vi "MES_Get Parameters.vi"(0 "Name":string, 1 "Order By":T1, 5 "Main":string, 9 "VariableName":string, 11 "error in (no error)":errorcluster, 12 "Alarm":bool=TRUE) -> (2 "FirstRow":string[](array[string]), 3 "Value1 List":string[](array[string]), 4 "Value 1":T2, 6 "Value  2":T2, 8 "Value  3":T2, 10 "Unit":string, 13 "First row value list":string[](array[string]), 14 "Table Control 2":string[][](table), 15 "error out":errorcluster)   [LabVIEW 2021, in "SQLite.lvclass"]
doc: "读取MES与PLC通讯的IP地址，DB块，DBB地址，format\n# 2020-5-13 13:25:16\n# daikinyi\n蒋松\njiangsong@outlook.com"
uses:
  SQLite.lvclass
  Control/value Type.ctl
  Order By.ctl
  TabelFullName.ctl
  SQLiteFileName.ctl
  <userlib>/LabSQL/LabSQL.lvlib
  <userlib>/sushu/sushu.lvlib
panel:
  out "formatList":string[](array[string])
  out "PLC DB DBBList":string[](array[string])
  out "number (0 to 1)":dbl
  out "Select SQL CMD":string
  # "组装线体的编号"
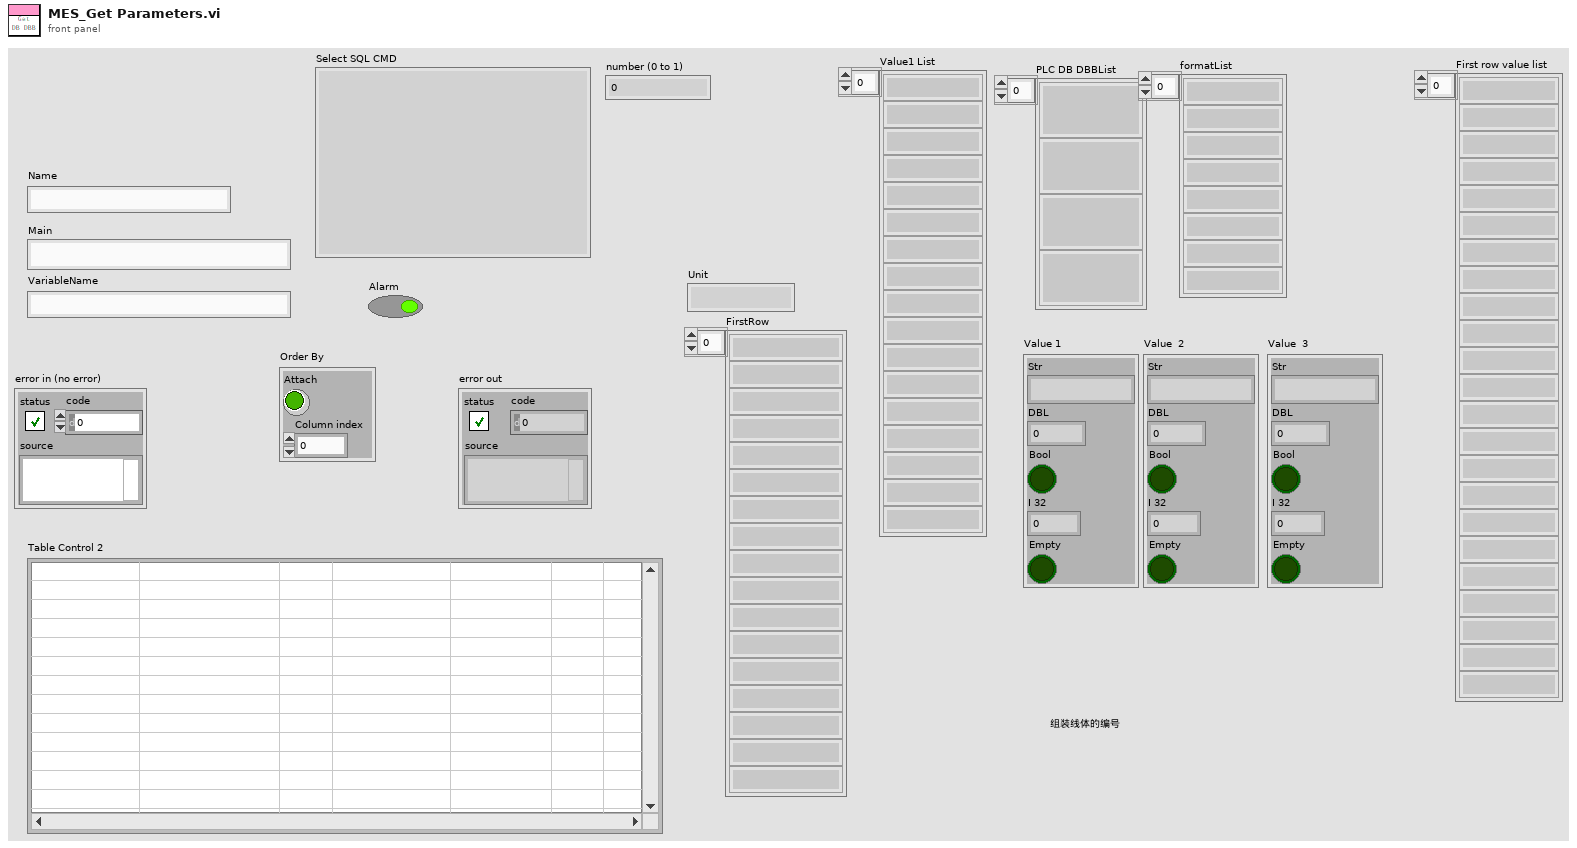
[diagram p1: front panel]
types:
  T1 = typedef "SQLite.lvclass/Order By.ctl" = cluster{"Attach":bool, "Column index":i32}
  T2 = typedef "SQLite.lvclass/value Type.ctl" = cluster{"Str":string, "DBL":dbl, "Bool":bool, "I 32":i32, "Empty":bool}
  T3 = enum16{"Initialize", "Read", "Write", "UnInitialize"}
  T4 = typedef "SQLite.lvclass/TabelFullName.ctl" = string
  T5 = cluster{"Current VI Reference":refnum<vi>, "Close Panel on Exit?":bool}
  T6 = cluster{"Core":cluster{"Current VI Reference":refnum<vi>, "Close Panel on Exit?":bool}, "VI Name":string}
  T7 = typedef "SQLite.lvclass/SQLiteFileName.ctl" = string
  T8 = enum16{"Other", "SQL2008", "SQLite", "Access", "MySQL"}
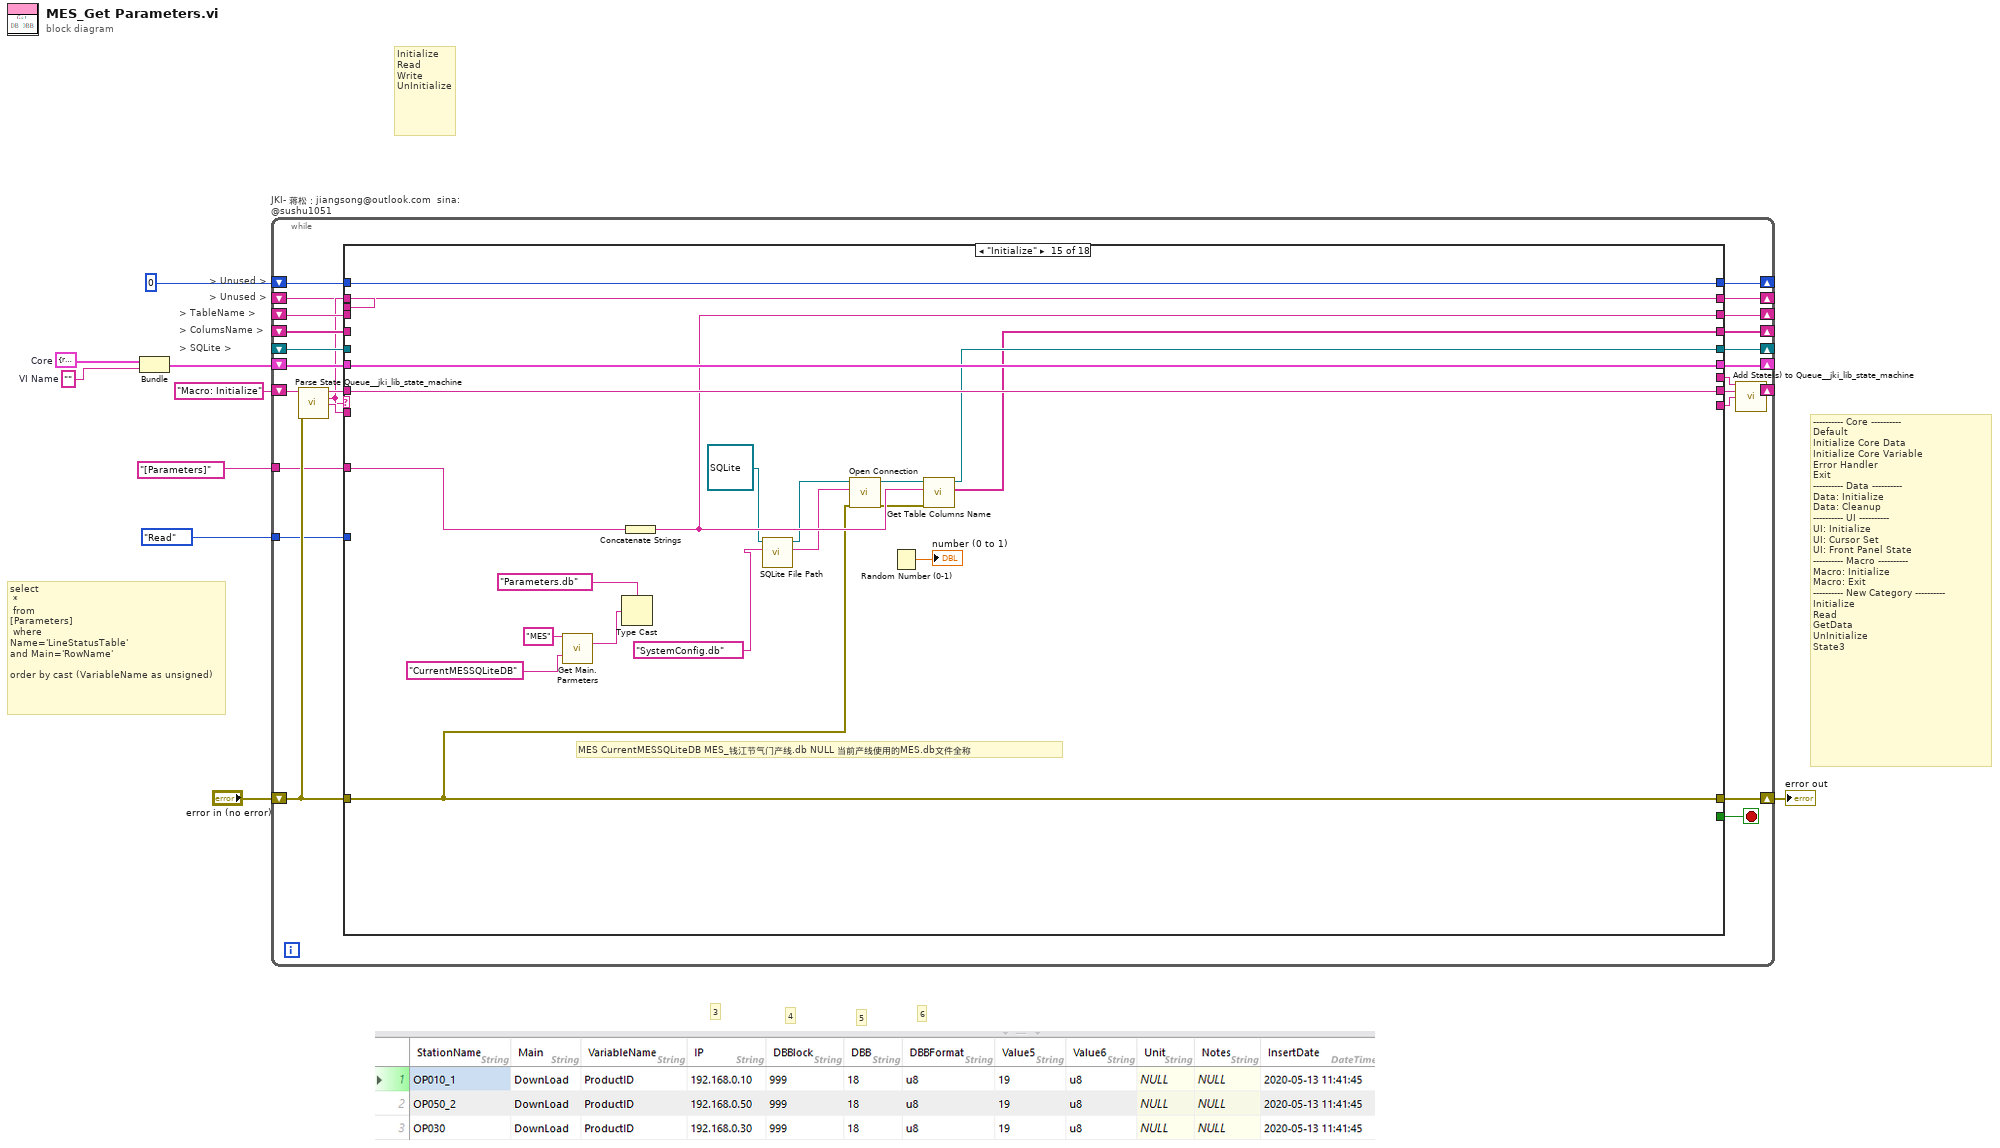
[diagram p0: block diagram]
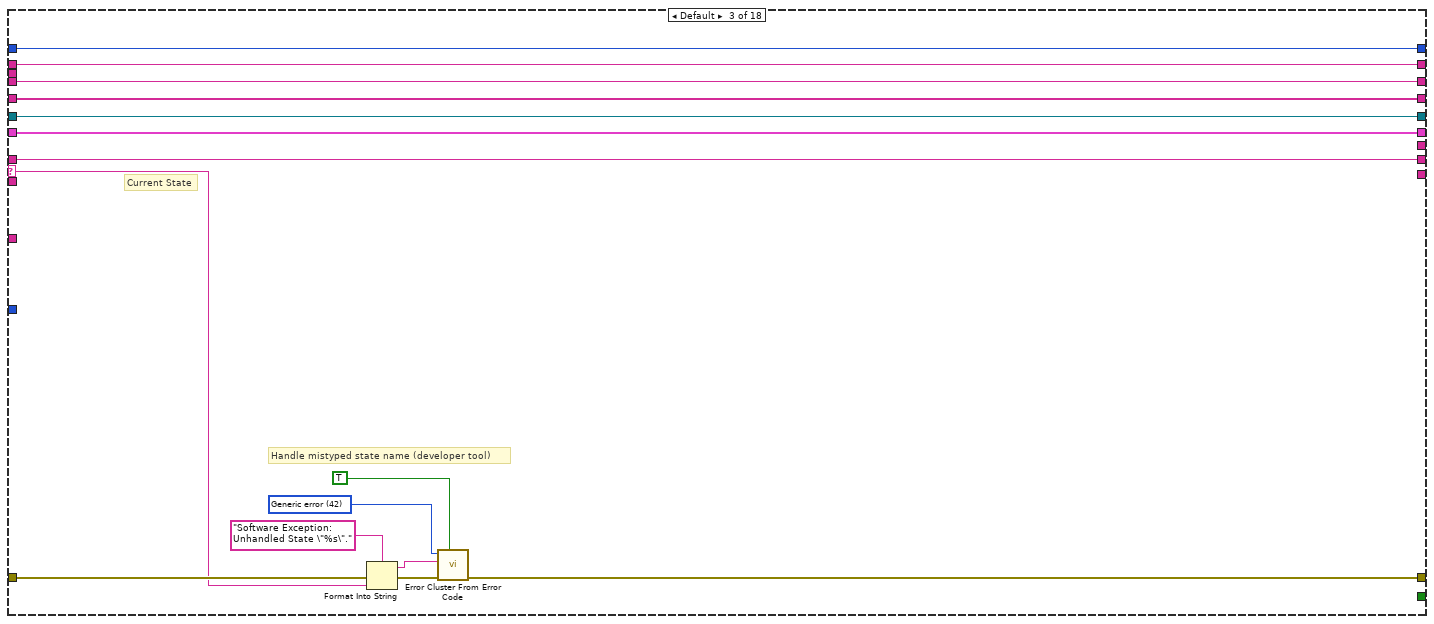
[diagram p4: hidden frame]
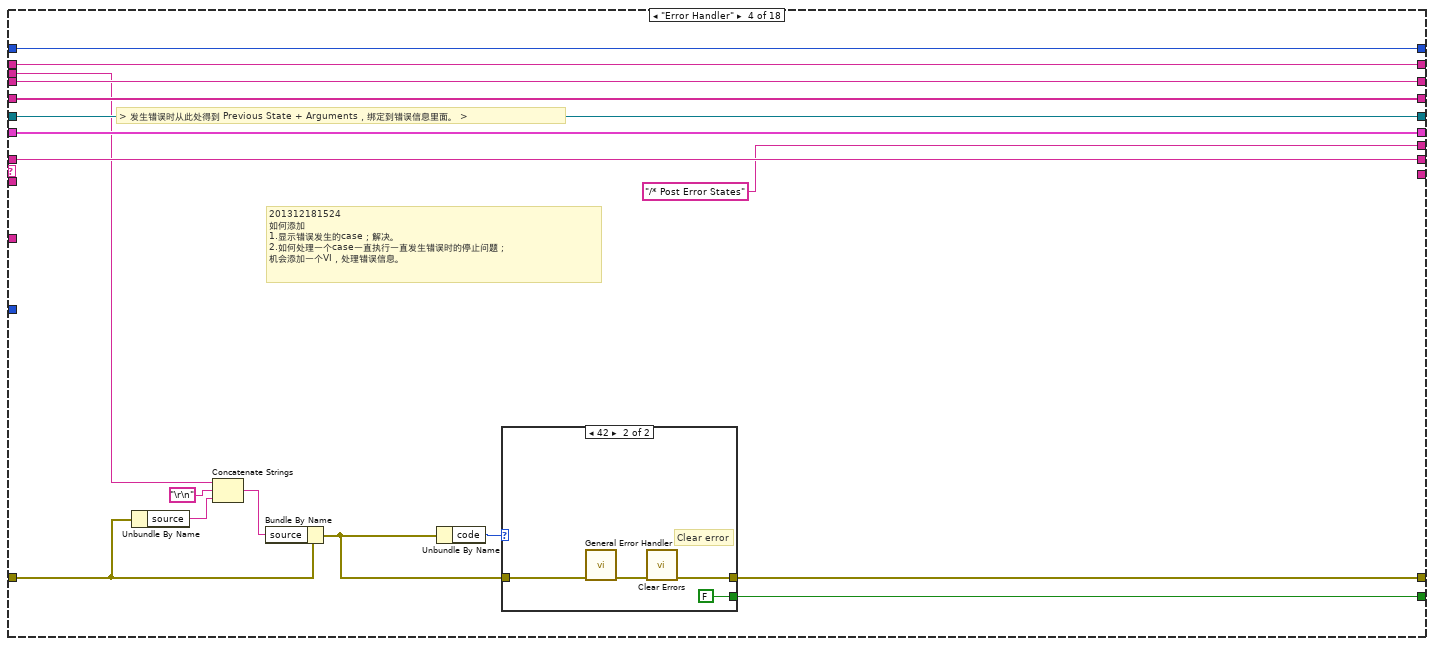
[diagram p5: hidden frame]
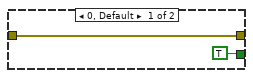
[diagram p6: hidden frame]
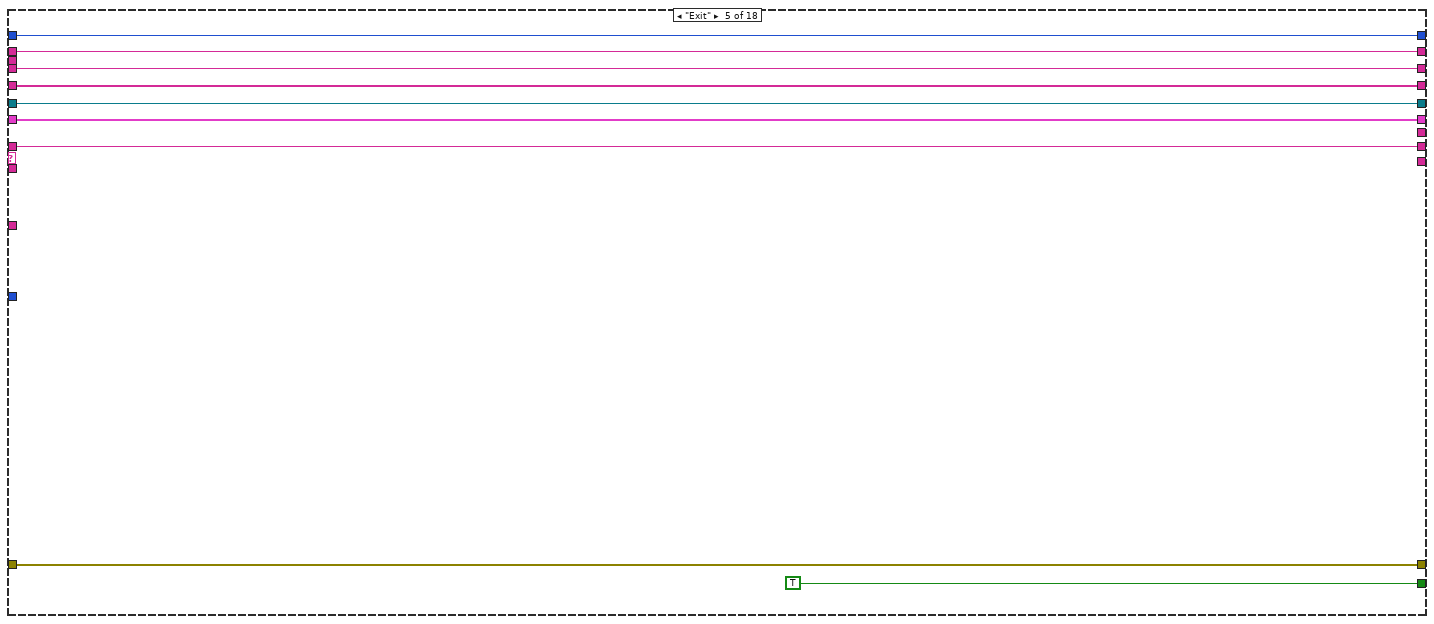
[diagram p7: hidden frame]
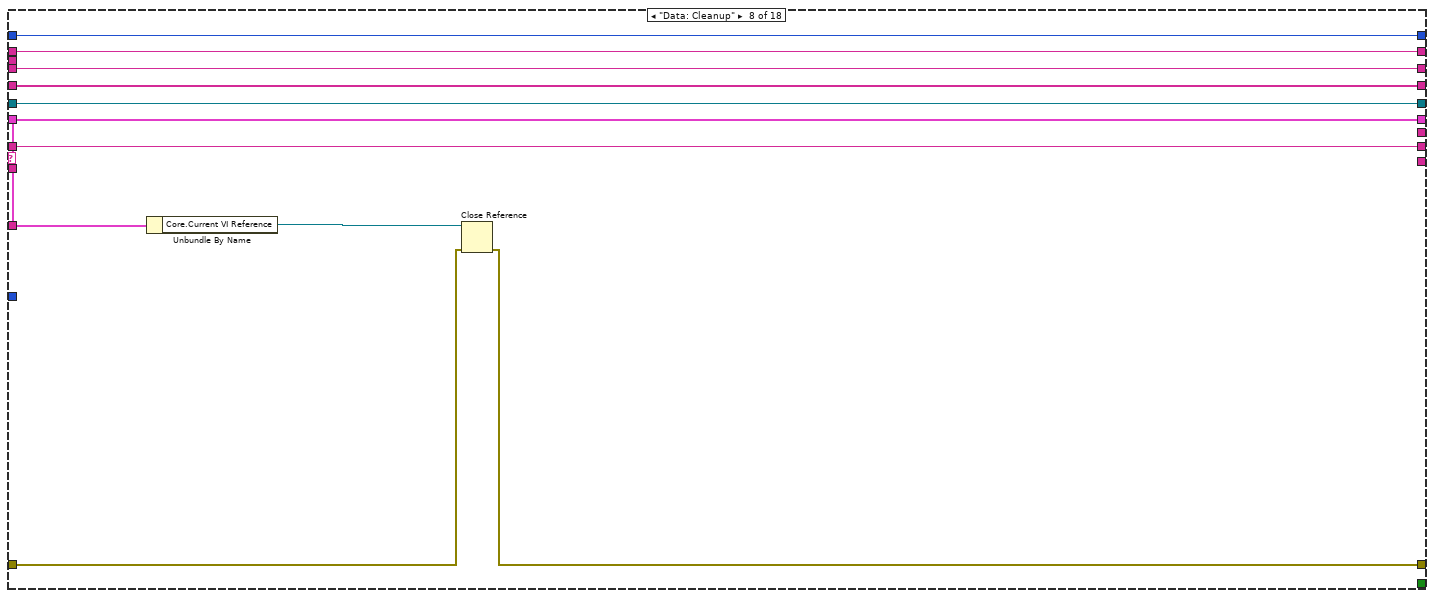
[diagram p10: hidden frame]
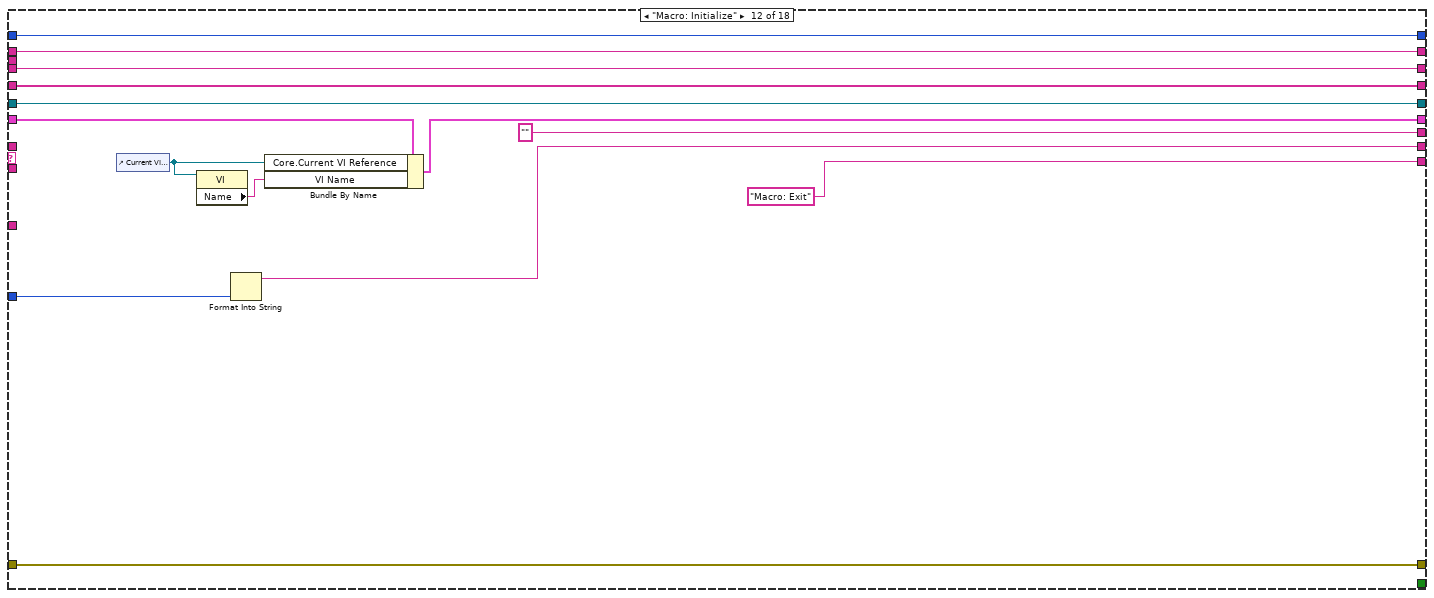
[diagram p14: hidden frame]
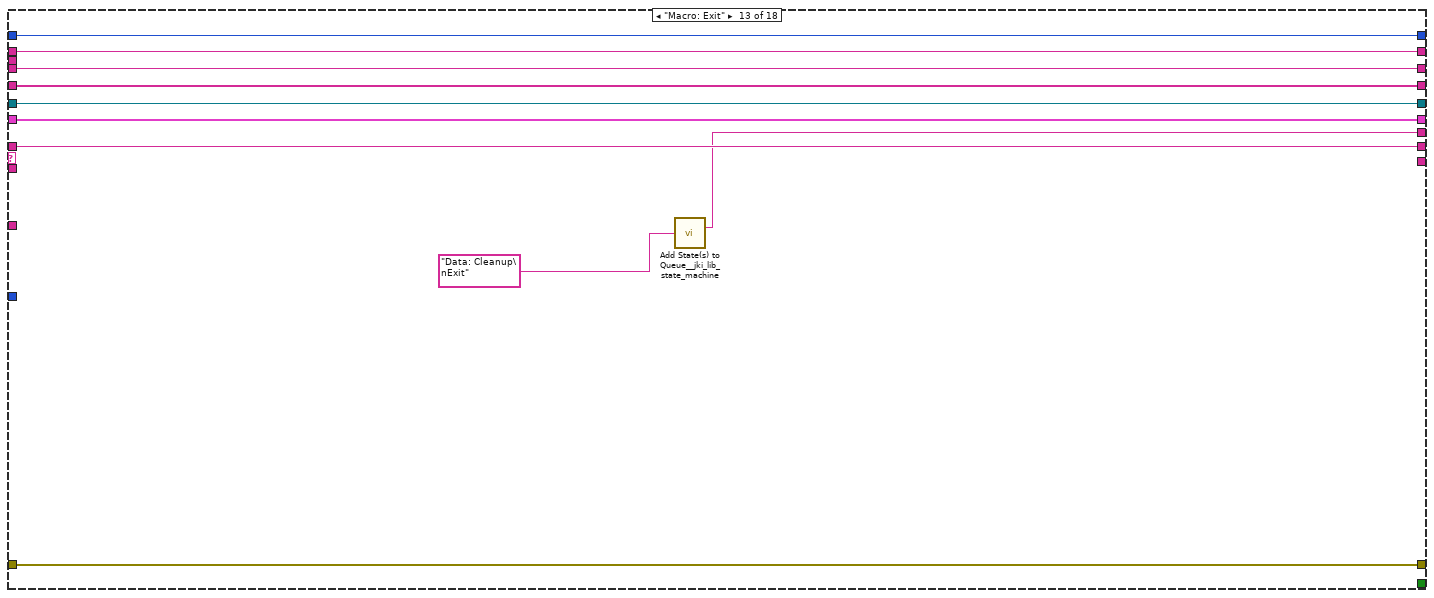
[diagram p15: hidden frame]
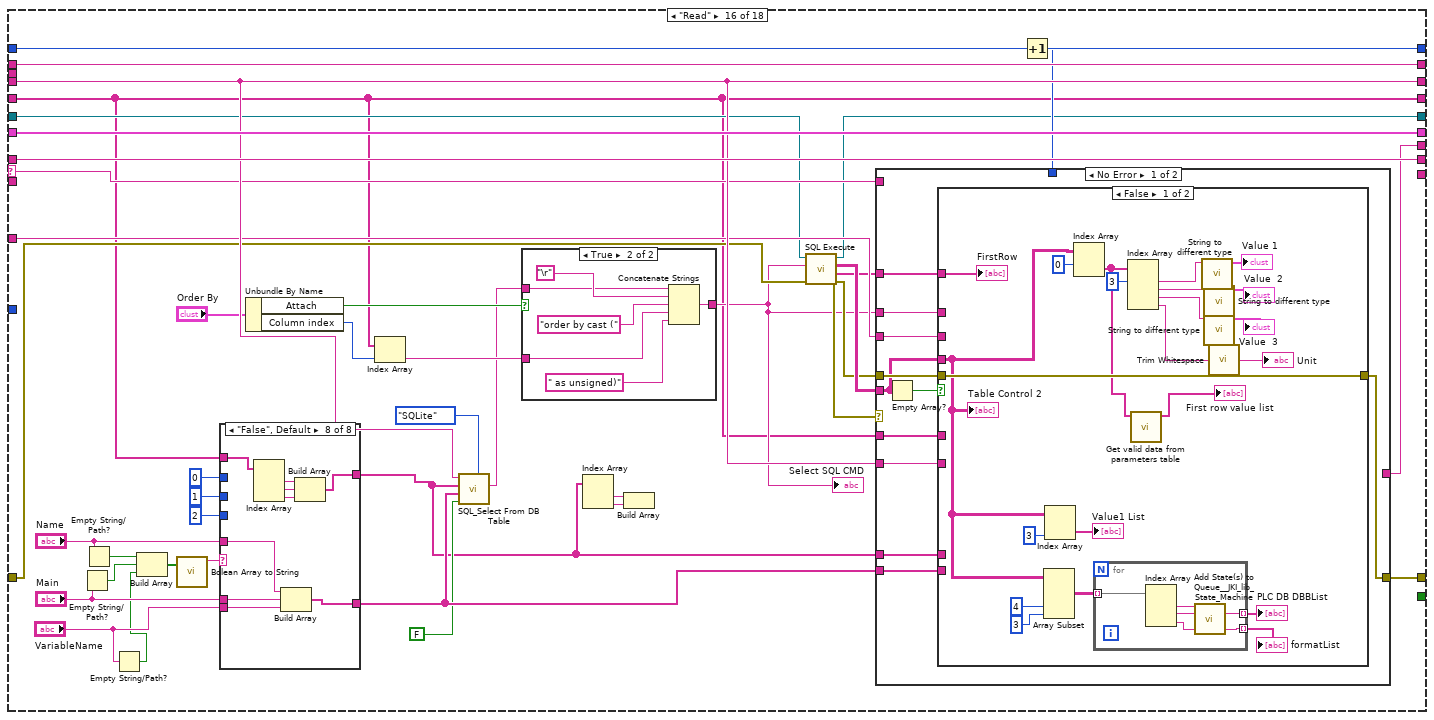
[diagram p17: hidden frame]
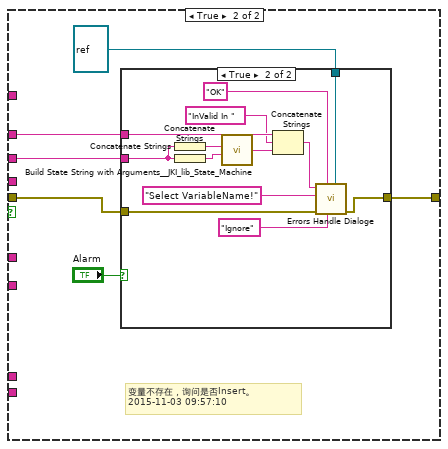
[diagram p19: hidden frame]
diagram:
  w9 = ""  # VI Name
  w8 = T5 {"Current VI Reference"=refnum, "Close Panel on Exit?"=FALSE}  # Core
  # "select \n * \n from \n[Parameters]\n where \nName='LineStatusTable'\nand Main='RowName'\n\norder by cast (VariableName as unsigned)"
  # "6"
  # "5"
  # "4"
  # "3"
  # "Initialize\nRead\nWrite\nUnInitialize"
  # "> Unused >"
  # "> SQLite >"
  # "> ColumsName >"
  # "> TableName >"
  # "> Unused >"
  # "---------- Core ----------\nDefault\nInitialize Core Data\nInitialize Core Variable\nError Handler\nExit\n---------- Data ----------\nData: Initialize\nData: Cleanup\n---------- UI ----------\nUI: Initialize\nUI: Cursor Set\nUI: Front Panel State\n---------- Macro ----------\nMacro: Initialize\nMacro: Exit\n---------- New Category ----------\nInitialize\nRead\nGetData\nUnInitialize\nState3"
  n1 = Bundle("Core"=w8, "VI Name"=w9) -> (w7:T6)  [unwired: 1 in]
  n2 = while "JKI- 蒋松：jiangsong@outlook.com  sina: @sushu1051" {
    shift-right: [w32] -> w2
    shift-left: "error in (no error)" -> [w30]
    shift-right: [w20] -> _
    shift-left: "Macro: Initialize" -> [w21]
    shift-right: [w27] -> _
    shift-left: _ -> [w29]
    shift-right: [w28] -> _
    shift-left: _ -> [w10]
    shift-right: [w22] -> _
    shift-left: w7 -> [w25]
    shift-right: [w23] -> _
    shift-left: _ -> [w16]
    shift-right: [w24] -> _
    shift-left: _ -> [w26]
    shift-right: [w15] -> _
    shift-left: 0 -> [w14]
    tunnel: T3."Read" ("CMD") -> [w13]
    tunnel: T4 "[Parameters]" ("TabelFullName") -> [w12]
    stop <- w31 stop-if-true
    n3 = call <vilib>:"Parse State Queue__jki_lib_state_machine.vi"("State Queue"=w21, "Error In (no error)"=w30) -> ("Remaining States"=w34:string, "Current State"=w11:string, "Arguments"=w33:string)  [unwired: 10 in, 1 out]
    n4 = case shown="\"Initialize\"" w11 {
      selector: w11 -> [_ _ w53 _ _ _ _ _ _ _ _ _ _ _ _ w230 _ _]
      tunnel: w34 -> [w42 w44 w52 w74 w90 w99 w108 w115 w125 w133 w141 _ w164 w173 w199 w239 w386 w396]
      tunnel: w33 -> [_ _ _ _ _ _ _ _ _ _ _ _ _ _ _ _ _ _]
      tunnel: [w41 w50 w54 w68 w92 w101 w110 w117 w127 w135 w143 w158 w168 w176 w189 w231 w379 w387] -> w32
      tunnel: w30 -> [w41 w50 w55 w78 w92 w101 w110 w118 w127 w135 w143 w158 w168 w176 w189 w224 w379 w388]
      tunnel: [w42 w44 w52 w74 w90 w99 w108 w115 w125 w133 w141 w149 w164 w173 w199 w239 w386 w396] -> w19
      tunnel: [_ _ _ w67 TRUE _ _ _ _ _ _ _ _ _ _ _ _ _] -> w31
      tunnel: w11 -> [w40 w49 w65 w82 w97 w105 w113 w123 w131 w139 w147 w161 w171 w179 w198 w232 w380 w395]
      tunnel: w29 -> [w39 w48 w64 w81 w96 w104 w112 w122 w130 w138 w146 w160 w170 w178 _ w234 w385 w394]
      tunnel: [w40 w49 w65 w82 w97 w105 w113 w123 w131 w139 w147 w161 w171 w179 w198 w232 w380 w395] -> w28
      tunnel: [w39 w48 w64 w81 w96 w104 w112 w122 w130 w138 w146 w160 w170 w178 w191 w234 w385 w394] -> w27
      tunnel: w26 -> [w38 w47 w63 w80 w95 w103 w111 w121 w129 w137 w145 w159 w169 w177 _ w206 w384 w393]
      tunnel: w16 -> [w36 w45 w62 w72 w91 w100 w109 w116 w126 w134 w142 w157 w165 w174 _ w227 w383 w390]
      tunnel: w25 -> [w37 w46 w61 w79 w94 w102 w106 w119 w128 w136 w144 w151 w166 w175 w197 w238 w382 w392]
      tunnel: [w38 w47 w63 w80 w95 w103 w111 w121 w129 w137 w145 w159 w169 w177 w192 w206 w384 w393] -> w24
      tunnel: [w36 w45 w62 w72 w91 w100 w109 w116 w126 w134 w142 w157 w165 w174 w193 w225 w383 w389] -> w23
      tunnel: [w37 w46 w61 w79 w94 w102 w106 w119 w128 w136 w144 w150 w166 w175 w197 w238 w382 w392] -> w22
      tunnel: [_ _ _ "/* Post Error States" _ _ _ _ _ _ _ "" w163 _ _ w229 _ _] -> w18
      tunnel: [_ _ _ _ _ _ _ _ _ _ _ "Macro: Exit" _ _ _ _ _ _] -> w17
      tunnel: w14 -> [w35 w43 w51 w71 w89 w98 w107 w114 w124 w132 w140 w156 w162 w172 w196 w228 w381 w391]
      tunnel: [w35 w43 w51 w71 w89 w98 w107 w114 w124 w132 w140 w156 w162 w172 w196 w237 w381 w391] -> w15
      tunnel: w13 -> [_ _ _ _ _ _ _ _ _ _ _ w148 _ _ _ _ _ _]
      tunnel: w12 -> [_ _ _ _ _ _ _ _ _ _ _ _ _ _ w194 w233 _ _]
      tunnel: w10 -> [_ _ _ w66 _ _ _ _ _ _ _ _ _ _ _ _ _ _]
      frame "Idle" {
      }
      frame "---------- Core ----------" {
      }
      frame Default {
        w57 = 42 items=["No error", "Argument error", "Memory is full", "Out of zone", "End of file", "File already open", "Generic file I/O error", "File not found", "File permission error", "Disk is full", "Duplicate path", "Too many files open", "System feature not enabled", "Resource file not found", "Cannot add resource", "Resource not found", "Image not found", "Image memory error", "Pen does not exist", "Config type invalid", "Config token not found", "Config parse error", "Config memory error", "Bad external code format", "Bad external code offset", "External code not present", "Null window", "Destroy window error", "Null menu", "Print aborted", "Bad print record", "Print driver error", "Windows error during printing", "Memory error during printing", "Print dialog error", "Generic print error", "Invalid device refnum", "Device not found", "Device parameter error", "Device unit error", "Cannot open device", "Device call aborted", "Generic error", "Cancelled by user", "Object ID too low", "Object ID too high", "Object not in heap", "Unknown heap", "Unknown object (invalid DefProc)", "Unknown object (DefProc not in table)", "Message out of range", "Invalid (null) method", "Unknown message", "Manager call not supported", "Bad address", "Network operation in progress", "Network operation timed out", "Connection is busy", "Network attribute not supported", "Network error", "Address in use", "System out of memory", "Connection aborted", "Connection refused", "Not connected", "Already connected", "Connection closed", "Initialization error (interapplication manager)", "Bad occurrence", "Wait on unbound occurrence handler", "Occurrence queue overflow", "Datalog type conflict", "Unused", "Unrecognized type (interapplication manager)", "Memory corrupt", "Failed to make temporary DLL", "Old CIN version", "Drag socket not found", "Failed to load drop-object", "Failed to register OLE object", "Failed to release OLE object", "Format specifier type mismatch", "Unknown format specifier", "Too few format specifiers", "Too many format specifiers", "Scan failed", "Newer CIN version", "Error converting to variant", "Runtime menu error", "Password tampered", "Variant attribute not found", "Incompatible variant data type", "Event data is not available", "Event Store is not present", "Occurrence is not found", "Event Queue is not created", "Event info is not available", "Refnum passed is NULL", "Error retrieving Class GUID", "Error retrieving CoClass GUID", "Error retrieving TypeLib GUID.", "Bad built application magic bytes.", "Specific driver is different from the specific driver associated with the Logical Name.", "There is no session opened to the class driver.", "Max Error", "MAX - Error with config objects", "MAX - Error loading configuration", "MAX - Group not supported"]
        # "Current State"
        # "Handle mistyped state name (developer tool)"
        n5 = Format Into String(format string="Software Exception: Unhandled State \"%s\"." ("message"), error in=w55, w53) -> (resulting string=w58:string, error out=w59:errorcluster)  [unwired: 1 in]
        n6 = call <vilib>:"Error Cluster From Error Code.vi"("show call chain? (False)"=TRUE, "error in (no error)"=w59, "error message (\"\")"=w58, "error code (0)"=w57) -> ("error out"=w54:errorcluster)  [unwired: 5 in]
      }
      frame "Error Handler" {
        # "> 发生错误时从此处得到 Previous State + Arguments，绑定到错误信息里面。 >"
        # "201312181524\n如何添加\n1.显示错误发生的case；解决。\n2.如何处理一个case一直执行一直发生错误时的停止问题；\n机会添加一个VI，处理错误信息。"
        # "Clear error"
        n7 = Unbundle By Name(w78) -> ("source"=w76:string)
        n8 = Concatenate Strings(w66, "\r\n", w76) -> (w75:string)
        n9 = Bundle By Name(cluster=w78, "source"=w75) -> (w69:errorcluster)
        n10 = Unbundle By Name(w69) -> ("code"=w70:i32)
        n11 = case shown="42" w70 {
          tunnel: [TRUE FALSE] -> w67
          tunnel: w69 -> [w84 w87]
          tunnel: [w84 w85] -> w68
          frame 0, Default {
          }
          frame 42 {
            n12 = call <vilib>:"General Error Handler.vi"("error in (no error)"=w87) -> ("error out"=w86:errorcluster)  [unwired: 10 in, 4 out]
            n13 = call <vilib>:"Clear Errors.vi"("error in (no error)"=w86) -> ("error out"=w85:errorcluster)  [unwired: 5 in, 1 out]
          }
        }
      }
      frame "Exit" {
      }
      frame "---------- Data ----------" {
      }
      frame "Data: Initialize" {
      }
      frame "Data: Cleanup" {
        n14 = Unbundle By Name(w119) -> ("Core.Current VI Reference"=w120:refnum<vi>)
        n15 = Close Reference(reference=w120, error in (no error)=w118) -> (error out=w117:errorcluster)
      }
      frame "---------- UI ----------" {
      }
      frame "UI: Initialize" {
      }
      frame "---------- Macro ----------" {
      }
      frame "Macro: Initialize" {
        n16 = control-ref of="Current VI Reference"() -> (w152:refnum<vi>)
        n17 = property class="VI"(reference=w152) -> ("Name"=w153:string)  [unwired: 1 in, 2 out]
        n18 = Format Into String(w148) -> (resulting string=w149:string)  [unwired: 3 in, 1 out]
        n19 = Bundle By Name(cluster=w151, "Core.Current VI Reference"=w152, "VI Name"=w153) -> (w150:T6)
      }
      frame "Macro: Exit" {
        n20 = call <vilib>:"Add State(s) to Queue__jki_lib_state_machine.vi"("State(s) at Back (\"\")"="Data: Cleanup\nExit") -> ("States Out"=w163:string)  [unwired: 14 in]
      }
      frame "---------- New Category ----------" {
      }
      frame "Initialize" {
        # "MES\tCurrentMESSQLiteDB\tMES_钱江节气门产线.db\tNULL\t当前产线使用的MES.db文件全称"
        n21 = call "Get Main.Parmeters.vi"("Main"="MES", "VariableName"="CurrentMESSQLiteDB" ("Main")) -> ("Value"=w182:string)  [unwired: 6 in, 7 out]
        n22 = Type Cast(type=T7 "Parameters.db" ("SQLiteFileName"), x=w182) -> ()  [unwired: 1 out]
        n23 = Concatenate Strings(w194) -> (w191:string)
        n24 = call "SQLite File Path.vi"("SQLiteFileName"=T7 "SystemConfig.db" ("*(type *) &x"), "SQLite in"=refnum<class "SQLite.lvclass"> refnum ("SQLite.lvclass")) -> ("string"=w188:string, "SQLite out"=w186:refnum<class "SQLite.lvclass">)  [unwired: 7 in, 1 out]
        n25 = call-dynamic "Open Connection.vi"("error in (no error)"=w189, "ConnectionString"=w188, "HostDB in"=w186) -> ("error out"=w190:errorcluster, "HostDB out"=w195:refnum<class "SQLite.lvclass">)  [unwired: 7 in]
        n26 = Random Number (0-1)() -> (number: 0 to 1=→"number (0 to 1)":dbl)
        n27 = call-dynamic "Get Table Columns Name.vi"("error in (no error)"=w190, "TableName"=w191, "HostDB in"=w195) -> ("Table_ColunmsList"=w192:string[], "HostDB out"=w193:refnum<class "SQLite.lvclass">)  [unwired: 4 in, 3 out]
      }
      frame "Read" {
        n28 = Empty String/Path?(string/path="Main") -> (empty?=w220:bool)
        n29 = Empty String/Path?(string/path="Name") -> (empty?=w221:bool)
        n30 = Empty String/Path?(string/path="VariableName") -> (empty?=w213:bool)
        n31 = Build Array(w221, w220, w213) -> (w219:bool[])
        n32 = call <userlib>:"Bolean Array to String.vi"("Bolean Array"=w219) -> ("Bolean String"=w218:string)  [unwired: 10 in]
        n33 = case shown="\"False\", Default" w218 {
          tunnel: [w327 w333 w334 w341 w350 w360 w369 w378] -> w236
          tunnel: "Main" -> [w326 _ _ _ w348 w358 _ w377]
          tunnel: "VariableName" -> [w325 w332 _ _ _ w357 w367 w376]
          tunnel: "Name" -> [_ _ _ w340 w349 w359 w368 w375]
          tunnel: w206 -> [w321 w330 _ w338 w345 w354 w366 w372]
          tunnel: 0 ("index") -> [_ _ _ w337 w344 w353 w363 _]
          tunnel: 2 ("index") -> [w319 w329 _ _ _ _ w362 _]
          tunnel: [w320 w328 w334 w336 w342 w351 w361 w370] -> w200
          tunnel: 1 ("index") -> [w322 _ _ _ w343 _ _ _]
          frame "100" {
            n34 = Index Array(array=w321, index #1=w322, index #2=w319) -> (element #1=w324:string, element #2=w323:string)
            n35 = Build Array(w326, w325) -> (w327:string[])
            n36 = Build Array(w324, w323) -> (w320:string[])
          }
          frame "110" {
            n37 = Index Array(array=w330, index #1=w329) -> (element #1=w331:string)  [unwired: 1 in, 1 out]
            n38 = Build Array(w332) -> (w333:string[])
            n39 = Build Array(w331) -> (w328:string[])
          }
          frame "111" {
            n40 = Build Array("" ("VariableName")) -> (w334:string[])
          }
          frame "011" {
            n41 = Index Array(array=w338, index #1=w337) -> (element #1=w339:string)  [unwired: 1 in, 1 out]
            n42 = Build Array(w340) -> (w341:string[])
            n43 = Build Array(w339) -> (w336:string[])
          }
          frame "001" {
            n44 = Build Array(w349, w348) -> (w350:string[])
            n45 = Index Array(array=w345, index #1=w344, index #2=w343) -> (element #1=w347:string, element #2=w346:string)
            n46 = Build Array(w347, w346) -> (w342:string[])
          }
          frame "000" {
            n47 = Index Array(array=w354, index #1=w353) -> (element #1=w356:string, element #2=w355:string, element #3=w352:string)  [unwired: 2 in]
            n48 = Build Array(w359, w358, w357) -> (w360:string[])
            n49 = Build Array(w356, w355, w352) -> (w351:string[])
          }
          frame "010" {
            n50 = Build Array(w368, w367) -> (w369:string[])
            n51 = Index Array(array=w366, index #1=w363, index #2=w362) -> (element #1=w365:string, element #2=w364:string)
            n52 = Build Array(w365, w364) -> (w361:string[])
          }
          frame "False", Default {
            n53 = Index Array(array=w372) -> (element #1=w374:string, element #2=w373:string, element #3=w371:string)  [unwired: 3 in]
            n54 = Build Array(w375, w377, w376) -> (w378:string[])
            n55 = Build Array(w374, w373, w371) -> (w370:string[])
          }
        }
        n56 = Unbundle By Name("Order By") -> ("Attach"=w211:bool, "Column index"=w210:i32)
        n57 = Index Array(array=w206, index=w210) -> (element=w212:string)
        n58 = call <userlib>:"SQL_Select From DB Table.vi"("DB Type"=T8."SQLite", "Check ASCII?"=FALSE, "ColumnsValue"=w236, "ColumnsNameList"=w200, "TableName"=w234) -> ("Select SQL CMD"=w208:string)  [unwired: 6 in]
        n59 = case shown="True" w211 {
          tunnel: w208 -> [w240 w245]
          tunnel: w212 -> [_ w243]
          tunnel: [w240 w241] -> w207
          frame False {
          }
          frame True {
            n60 = Concatenate Strings(w245, "\r", "order by cast (" ("string"), w243, " as unsigned)" ("string")) -> (w241:string)
          }
        }
        "Select SQL CMD" <- w207
        n61 = Index Array(array=w200) -> (element #1=w201:string, element #2=w202:string)  [unwired: 2 in]
        n62 = Build Array(w201, w202) -> ()  [unwired: 1 out]
        n63 = call-dynamic "SQL Execute.vi"("error in (no error)"=w224, "Command Text"=w207, "HostDB in"=w227) -> ("error out"=w223:errorcluster, "FirstRow"=w216:string[], "Table Control"=w226:string[][], "HostDB out"=w225:refnum<class "SQLite.lvclass">)  [unwired: 4 in, 1 out]
        n64 = case shown="No Error" w223 {
          selector: w223 -> [_ w308]
          tunnel: w200 -> [w257 _]
          tunnel: w223 -> [w256 w318]
          tunnel: w207 -> [w254 _]
          tunnel: w226 -> [w253 _]
          tunnel: w236 -> [w252 _]
          tunnel: w206 -> [w251 _]
          tunnel: w234 -> [w250 _]
          tunnel: w233 -> [w249 _]
          tunnel: [w248 w317] -> w231
          tunnel: w230 -> [_ w307]
          tunnel: [_ w306] -> w229
          tunnel: w228 -> [_ w305]
          tunnel: w216 -> [w247 _]
          frame No Error {
            n65 = Empty Array?(array=w253) -> (empty?=w255:bool)
            n66 = case shown="False" w255 {
              tunnel: [w279 w289] -> w248
              tunnel: w251 -> [_ _]
              tunnel: w250 -> [_ _]
              tunnel: w252 -> [_ _]
              tunnel: w257 -> [_ _]
              tunnel: w256 -> [w279 w290]
              tunnel: w254 -> [_ w287]
              tunnel: w249 -> [_ w288]
              tunnel: w253 -> [w260 _]
              tunnel: w247 -> [w267 _]
              frame False {
                n67 = Array Subset(array=w260, index (col)=4 ("index"), length (col)=3 ("length")) -> (w270:string[][])  [unwired: 2 in]
                n68 = Index Array(array=w260, index (col)=3 ("disabled index (col)")) -> (element=→"Value1 List":string[])  [unwired: 1 in]
                n69 = Index Array(array=w260, index (row)=0) -> (element=w259:string[])  [unwired: 1 in]
                n70 = for {
                  tunnel: w270 -> [w284] mode=indexing
                  tunnel: [w281] -> w269 mode=indexing
                  tunnel: [w280] -> w268 mode=indexing
                  n71 = Index Array(array=w284) -> (element #1=w283:string, element #2=w282:string, element #3=w280:string)  [unwired: 3 in]
                  n72 = call <vilib>:"Add State(s) to Queue__JKI_lib_State_Machine.vi"("State(s) in Front (\"\")"=w283, "State(s) in (\"\")"=w282) -> ("States Out"=w281:string)  [unwired: 13 in]
                }
                "PLC DB DBBList" <- w269
                "formatList" <- w268
                n73 = Index Array(array=w259, index #1=3 ("index")) -> (element #1=w266:string, element #2=w265:string, element #3=w264:string, element #4=w275:string)  [unwired: 3 in]
                n74 = call "Get valid data from parameters table.vi"("Parameter Full Row Data"=w259) -> ("array w/ subset deleted"=→"First row value list":string[])  [unwired: 10 in]
                n75 = call "String to different type.vi"("Value"=w266) -> ("Value"=→"Value 1":T2)  [unwired: 10 in]
                n76 = call "String to different type.vi"("Value"=w265) -> ("Value"=→"Value  2":T2)  [unwired: 10 in]
                n77 = call "String to different type.vi"("Value"=w264) -> ("Value"=→"Value  3":T2)  [unwired: 10 in]
                n78 = call <vilib>:"Trim Whitespace.vi"("string"=w275) -> ("trimmed string"=→"Unit":string)  [unwired: 1 in]
                "FirstRow" <- w267
                "Table Control 2" <- w260
              }
              frame True {
                # "变量不存在，询问是否Insert。\n2015-11-03 09:57:10"
                n79 = case shown="True" "Alarm" {
                  tunnel: w290 -> [w291 w304]
                  tunnel: [w291 w303] -> w289
                  tunnel: w288 -> [_ w292]
                  tunnel: w287 -> [_ w302]
                  tunnel: refnum<vi> refnum ("VI Ref") -> [_ w293]
                  frame False {
                  }
                  frame True {
                    n80 = Concatenate Strings(w292) -> (w301:string)
                    n81 = Concatenate Strings(w292) -> (w300:string)
                    n82 = call <vilib>:"Build State String with Arguments__JKI_lib_State_Machine.vi"("Arguments (\"\")"=w300, "State"=w301) -> ("State with Arguments"=w298:string)  [unwired: 4 in]
                    n83 = Concatenate Strings(w302, "InValid In " ("Message"), w298) -> (w297:string)
                    n84 = call <userlib>:"Errors Handle Dialoge.vi"("VI Ref"=w293, "Cancel Text"="Ignore", "OK Text"="OK", "error in (no error)"=w304, "Title Text"="Select VariableName!", "Message"=w297) -> ("error out"=w303:errorcluster)  [unwired: 4 in, 1 out]
                  }
                }
              }
            }
          }
          frame Error {
            n85 = call <vilib>:"Clear Errors.vi"("error in (no error)"=w318) -> ("error out"=w317:errorcluster)  [unwired: 5 in, 1 out]
            n86 = Unbundle By Name(w308) -> ("code"=w315:i32)
            n87 = Equal?(x=w315, y=7) -> (x = y?=w313:bool)
            n88 = Equal To 0?(x=w305) -> (x = 0?=w312:bool)
            n89 = And(x=w313, y=w312) -> (x .and. y?=w311:bool)
            n90 = call <vilib>:"Add State(s) to Queue__jki_lib_state_machine.vi"("State(s) in Front (\"\")"="Initialize" ("Remaining States"), "State(s) in (\"\")"=w307) -> ("States Out"=w309:string)  [unwired: 13 in]
            n91 = Select(t=w309, s=w311, f="GetData") -> (s? t:f=w306:string)
          }
        }
        n92 = Increment(x=w228) -> (x+1=w237:i32)
      }
      frame "GetData" {
      }
      frame "UnInitialize" {
        n93 = call-dynamic "Close Connection.vi"("error in (no error)"=w388, "HostDB in"=w390) -> ("error out"=w387:errorcluster, "HostDB out"=w389:refnum<class "SQLite.lvclass">)  [unwired: 8 in]
      }
    }
    n94 = call <vilib>:"Add State(s) to Queue__jki_lib_state_machine.vi"("State(s) in Front (\"\")"=w18, "State(s) in (\"\")"=w19, "State(s) at Back (\"\")"=w17) -> ("States Out"=w20:string)  [unwired: 12 in]
  }
  "error out" <- w2
